vi "GenerateGaussianBeamImage.vi"(8 "error in (no error)":errorcluster, 9 "Image Resolution":cluster{"X Step":u16, "Y Step":u16}={"X Step"=1280, "Y Step"=1024}, 10 "Fits Pixel":dbl[](array[numeric]), 11 "Image":T1) -> (0 "error out":errorcluster, 3 "Gaussian Surface Image":T1(plugin-control))   [LabVIEW 2015]
uses:
  <vilib>/vision/Image Controls.llb/IMAQ Image.ctl
panel:
  # "Amplitude"
  # "Position Mean X"
  # "Position Mean Y"
  # "Width 1"
  # "Width 2"
  # "Orient. Angle"
  # "Offset"
  # "x"
  # "pixels"
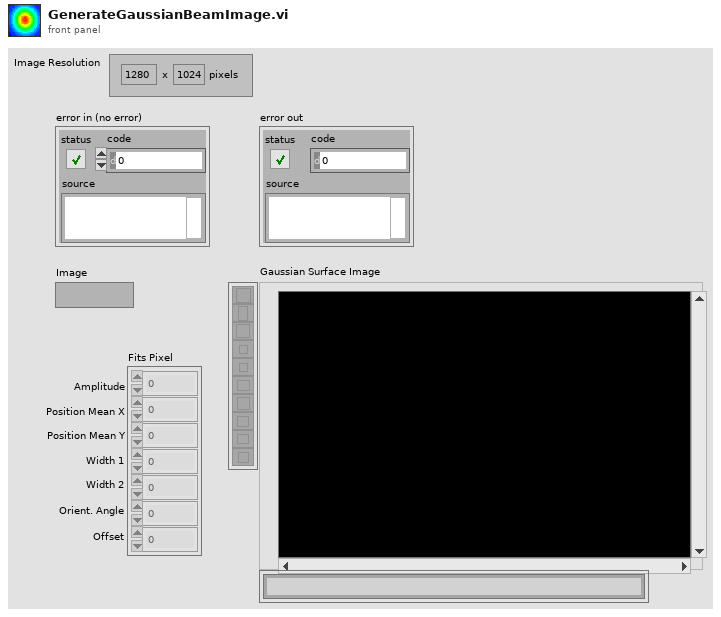
[diagram p1: front panel]
types:
  T1 = typedef "IMAQ Image.ctl" = refnum<image>
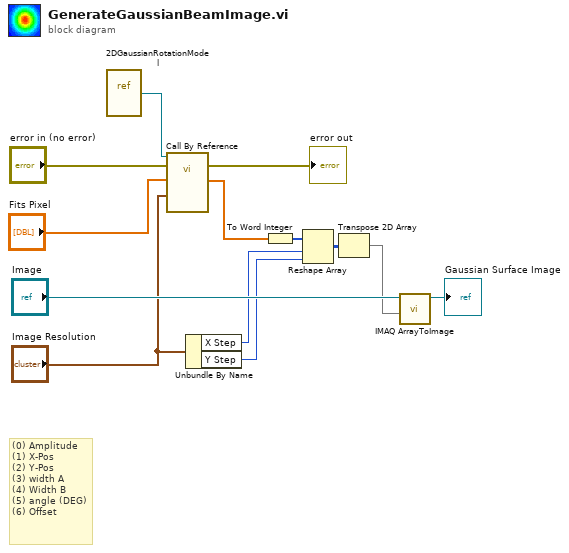
[diagram p0: block diagram]
diagram:
  # "(0) Amplitude\n(1) X-Pos\n(2) Y-Pos\n(3) width A\n(4) Width B\n(5) angle (DEG)\n(6) Offset"
  n1 = vi-ref "2DGaussianRotationModel.vi"() -> (w13:refnum<vi>)
  n2 = call-by-ref "?"(reference=w13, error in="error in (no error)", "data"="Image Resolution", "a"="Fits Pixel") -> (error out=→"error out":errorcluster, "f(X,a)"=w5:dbl[])  [unwired: 2 in, 3 out]
  n3 = Unbundle By Name("Image Resolution") -> ("X Step"=w2:u16, "Y Step"=w1:u16)
  n4 = To Word Integer(number=w5) -> (16bit integer=w7:i16[])
  n5 = Reshape Array(w7, w2, w1) -> (w8:i16[][])
  n6 = Transpose 2D Array(2D array=w8) -> (transposed array=w4:i16[][])
  n7 = call "IMAQ ArrayToImage"("Image Pixels (I16)"=w4, "Image"="Image") -> ("Image Out"=→"Gaussian Surface Image":T1)  [unwired: 8 in, 1 out]
